vi "Refresh Table.vi"(6 "IsCalibration":bool, 7 "Limit Status":T1, 8 "error in":errorcluster, 9 "Data String":string[][](array[string]), 10 "Col Header String":string[](array[string]), 11 "Result Table":refnum<vi>) -> (0 "error out":errorcluster, 1 "Data String dup":string[][](array[string]), 2 "Col Header String dup":string[](array[string]), 3 "Result Table dup":refnum<vi>)   [LabVIEW 2020, in "GUCalibration2.lvlib"]
uses:
  GUCalibration2.lvlib
  <vilib>/Utility/miscctls.llb/LVRowAndColumnTypeDef.ctl
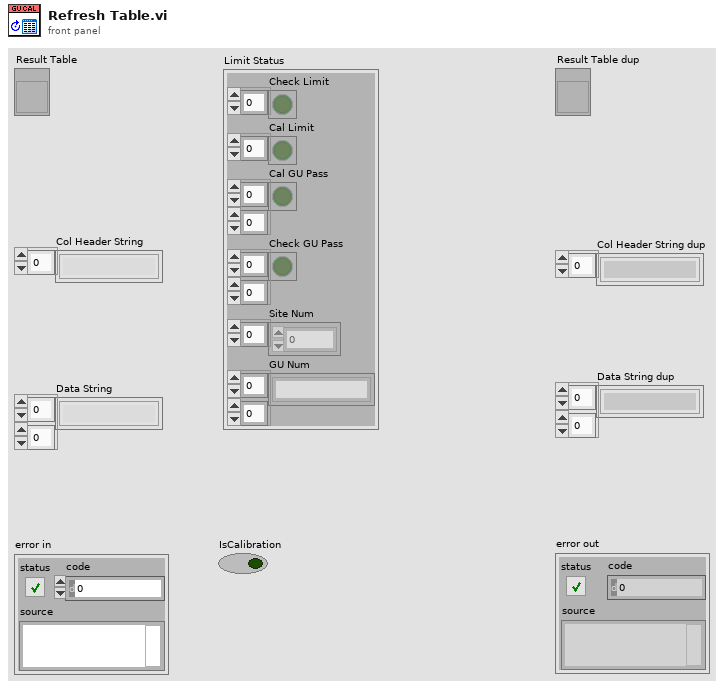
[diagram p1: front panel]
types:
  T1 = cluster{"Check Limit":bool[], "Cal Limit":bool[], "Cal GU Pass":bool[][], "Check GU Pass":bool[][], "Site Num":i32[], "GU Num":string[][]}
  T2 = typedef "LVRowAndColumnTypeDef.ctl" = cluster{"Row":i32, "Column":i32}
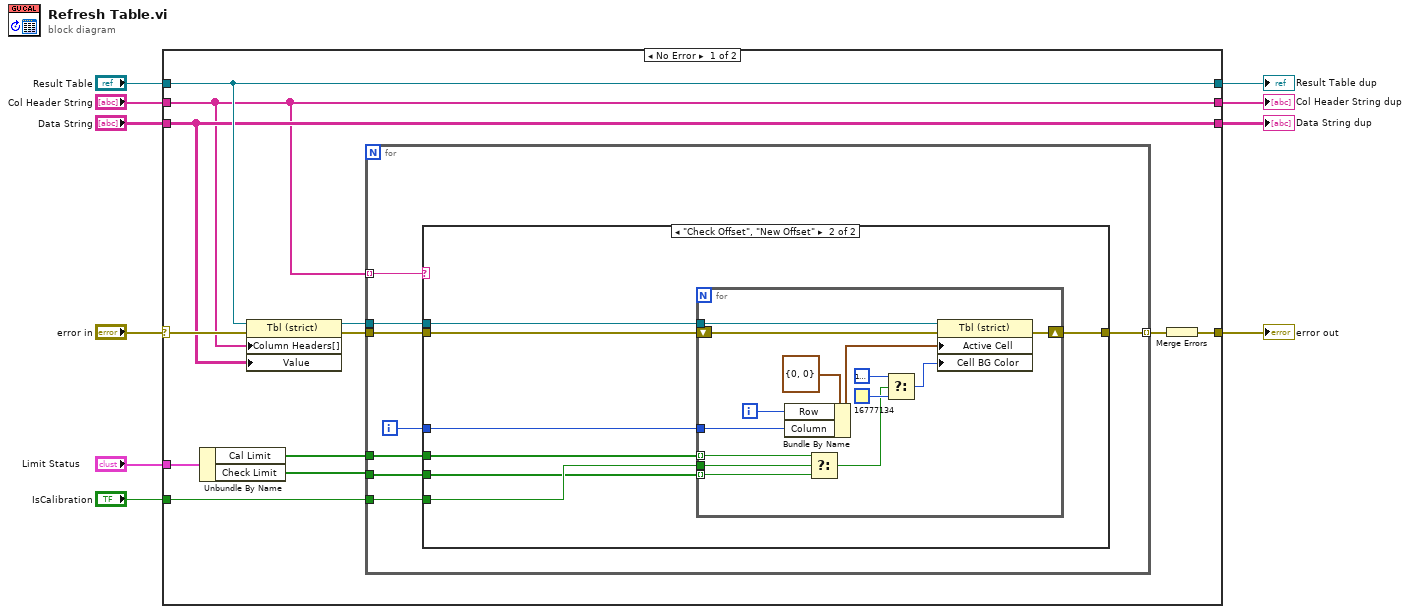
[diagram p0: block diagram]
diagram:
  n1 = case shown="No Error" "error in" {
    selector: "error in" -> [w18 w56]
    tunnel: "Result Table" -> [w17 w55]
    tunnel: "Col Header String" -> [w14 w54]
    tunnel: "Data String" -> [w16 w53]
    tunnel: [w19 w56] -> w8
    tunnel: [w17 w55] -> w6
    tunnel: [w14 w54] -> w5
    tunnel: [w16 w53] -> w4
    tunnel: "IsCalibration" -> [w15 _]
    tunnel: "Limit Status" -> [w13 _]
    frame No Error {
      n2 = Unbundle By Name(w13) -> ("Cal Limit"=w12:bool[], "Check Limit"=w11:bool[])
      n3 = property class="Tbl (strict)"(reference=w17, error in=w18, "Column Headers[]"=w14, "Value"=w16) -> (reference out=w21:refnum<vi>, error out=w22:errorcluster)
      n4 = for {
        tunnel: w22 -> [w27]
        tunnel: w21 -> [w28]
        tunnel: w14 -> [w30] mode=indexing
        tunnel: [w26] -> w20 mode=indexing
        tunnel: w15 -> [w25]
        tunnel: w12 -> [w24]
        tunnel: w11 -> [w23]
        i -> [w29]
        n5 = case shown="\"Check Offset\", \"New Offset\"" w30 {
          tunnel: w29 -> [_ w36]
          tunnel: w28 -> [_ w38]
          tunnel: w27 -> [w31 w37]
          tunnel: [w31 w35] -> w26
          tunnel: w25 -> [_ w34]
          tunnel: w24 -> [_ w33]
          tunnel: w23 -> [_ w32]
          frame "", Default {
          }
          frame "Check Offset", "New Offset" {
            n6 = for {
              tunnel: w38 -> [w52]
              tunnel: w36 -> [w47]
              shift-right: [w46] -> w35
              shift-left: w37 -> [w51]
              tunnel: w33 -> [w40] mode=indexing
              tunnel: w34 -> [w42]
              tunnel: w32 -> [w39] mode=indexing
              i -> [w48]
              n7 = Bundle By Name(cluster=T2 {"Row"=0, "Column"=0} ("Active Cell:Active Cell"), "Row"=w48, "Column"=w47) -> (w49:T2)
              n8 = Select(t=w40, s=w42, f=w39) -> (s? t:f=w41:bool)
              n9 = Select(t=u32 16777225, s=w41, f=u32 16777134) -> (s? t:f=w43:u32)
              n10 = property class="Tbl (strict)"(reference=w52, error in=w51, "Active Cell"=w49, "Cell BG Color"=w43) -> (error out=w46:errorcluster)  [unwired: 1 out]
            }
          }
        }
      }
      n11 = Merge Errors(w20) -> (w19:errorcluster)
    }
    frame Error {
    }
  }
  "error out" <- w8
  "Result Table dup" <- w6
  "Col Header String dup" <- w5
  "Data String dup" <- w4
